vi "Lift Re-index Values.vi"(6 "Current Lower Value":dbl, 8 "Initial Upper Value":dbl, 9 "Initial Lower Value":dbl, 10 "Input for Re-indexing":dbl, 11 "Limit Switches":T5) -> (3 "Re-indexed Value":dbl)   [LabVIEW 2014]
uses:
  <vilib>/Rock Robotics/WPI/Switch/WPI_SwitchDevRef.ctl
  <vilib>/Rock Robotics/SystemInterfaces/DIO/FPGA_DIOChannel.ctl
  <vilib>/Rock Robotics/SystemInterfaces/Typedef/FPGA_TypedefDigitalModule.ctl
  <vilib>/Rock Robotics/SystemInterfaces/Counter/FPGA_CounterCtrSystemIndex.ctl
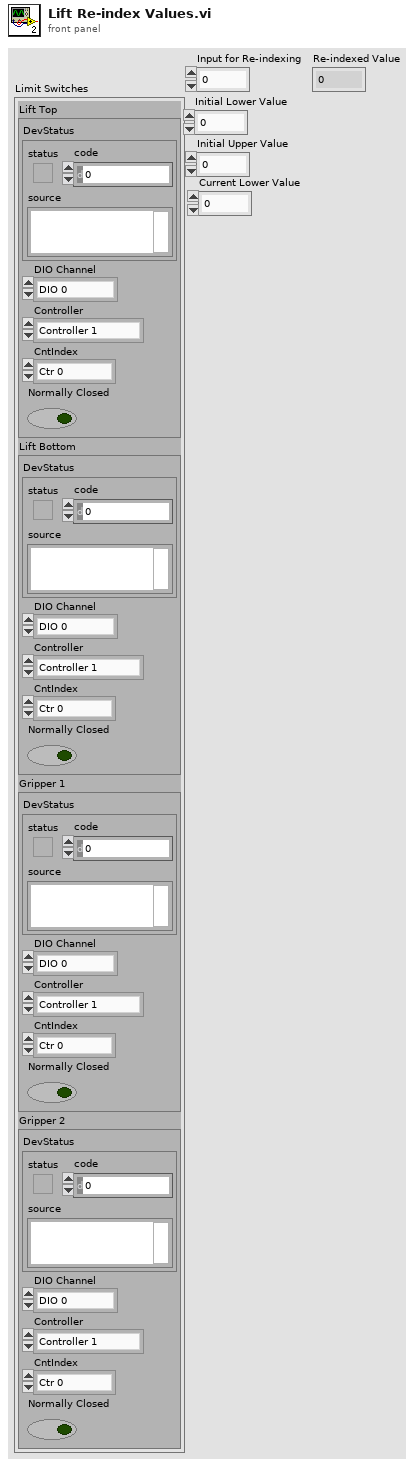
[diagram p1: front panel]
types:
  T1 = typedef "WPI_SwitchDevRef.ctl" = cluster{"DevStatus":errorcluster, "DIO Channel":T2, "Controller":T3, "CntIndex":T4, "Normally Closed":bool}
  T2 = typedef "FPGA_DIOChannel.ctl" = enum8{"DIO 0", "DIO 1", "DIO 2", "DIO 3", "DIO 4", "DIO 5", "DIO 6", "DIO 7", "DIO 8", "DIO 9", "DIO MXP 0", "DIO MXP 1", "DIO MXP 2", "DIO MXP 3", "DIO MXP 4", "DIO MXP 5", "DIO MXP 6", "DIO MXP 7", "DIO MXP 8", "DIO MXP 9", "DIO MXP 10", "DIO MXP 11", "DIO MXP 12", "DIO MXP 13", "DIO MXP 14", "DIO MXP 15", "Invalid"}
  T3 = typedef "FPGA_TypedefDigitalModule.ctl" = enum16{"Controller 1"}
  T4 = typedef "FPGA_CounterCtrSystemIndex.ctl" = enum8{"Ctr 0", "Ctr 1", "Ctr 2", "Ctr 3", "Ctr 4", "Ctr 5", "Ctr 6", "Ctr 7", "Invalid"}
  T5 = cluster{"Lift Top":T1, "Lift Bottom":T1, "Gripper 1":T1, "Gripper 2":T1}
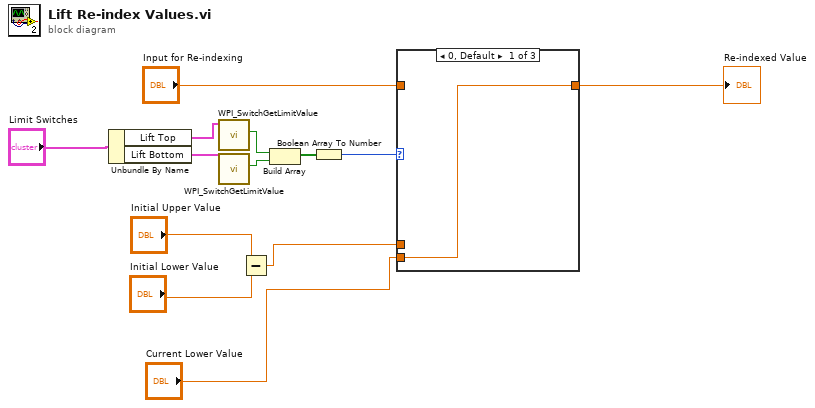
[diagram p0: block diagram]
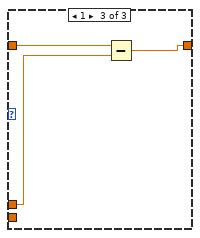
[diagram p3: hidden frame]
diagram:
  n1 = Unbundle By Name("Limit Switches") -> ("Lift Top"=w12:T1, "Lift Bottom"=w13:T1)
  n2 = call <vilib>:"WPI_SwitchGetLimitValue.vi"("SwitchDevRef"=w12) -> ("Switch Pressed"=w10:bool)  [unwired: 8 in, 2 out]
  n3 = call <vilib>:"WPI_SwitchGetLimitValue.vi"("SwitchDevRef"=w13) -> ("Switch Pressed"=w8:bool)  [unwired: 8 in, 2 out]
  n4 = Subtract(x="Initial Upper Value", y="Initial Lower Value") -> (x-y=w3:dbl)
  n5 = Build Array(w10, w8) -> (w9:bool[])
  n6 = Boolean Array To Number(Boolean array=w9) -> (number=w7:u32)
  n7 = case shown="0, Default" w7 {
    tunnel: "Input for Re-indexing" -> [_ w15 w17]
    tunnel: [w14 w15 w18] -> w5
    tunnel: w3 -> [_ _ w16]
    tunnel: "Current Lower Value" -> [w14 _ _]
    frame 0, Default {
    }
    frame 2 {
    }
    frame 1 {
      n8 = Subtract(x=w17, y=w16) -> (x-y=w18:dbl)
    }
  }
  "Re-indexed Value" <- w5
